vi "Detect Barcode.vi"() -> ()   [LabVIEW 2020]
doc: "Demonstrate the Barcode Detector"
uses:
  feature_detection/Barcode Detector/Detection.ctl
  feature_detection/Barcode Detector/Detection Region.ctl
  common/Image Point (Integer).ctl
  feature_detection/Barcode Detector/Barcode Detector.lvclass/Barcode Detector.ctl
  image/ARGB Colour.ctl
  image/Text Drawing Settings.ctl
  image/Font Face.ctl
  image/New Image (ARGB Preallocated).vi
  image/Copy Pixmap to Image (ARGB Flatten Mask).vi
  feature_detection/Barcode Detector/Detect Barcodes (ARGB).vi
  image/Draw Poly Lines (ARGB).vi
  image/Draw Text (ARGB).vi
  image/Draw Image to Picture (ARGB).vi
  image/New Image (ARGB Preallocated).vi/3321fa97-f432-4e1e-8db9-a0df79aed21b.vi
  image/ARGB Colour to U32 Pixel Value.vi
  image/Copy Pixmap to Image (ARGB Flatten Mask).vi/7d03ccf7-b889-4e8d-9f2a-57831e73dbde.vi
  feature_detection/Barcode Detector/Detect Barcodes (ARGB).vi/5cbfdd98-1063-43fc-ab47-121d1b6d8619.vi
  image/Draw Poly Lines (ARGB).vi/f4fe866f-059f-471d-887d-2797bd4b3b13.vi
  image/Draw Text (ARGB).vi/0015c4fc-6a12-4f82-815b-6c2f827f408b.vi
  image/Draw Image to Picture (ARGB).vi/8cd07b1b-062e-4fe4-9e87-2eb3dc89fe0e.vi
  image/FixPixmap.vi
  image/Default8bitColourMap.vi
  <vilib>/Utility/error.llb/Error Cluster From Error Code.vi
  image/image.lvlib
  feature_detection/Barcode Detector/Barcode Detector.lvclass
  common/common.lvlib
panel:
  out "Detections":T1[](array[typedef])
  out "Picture":picture
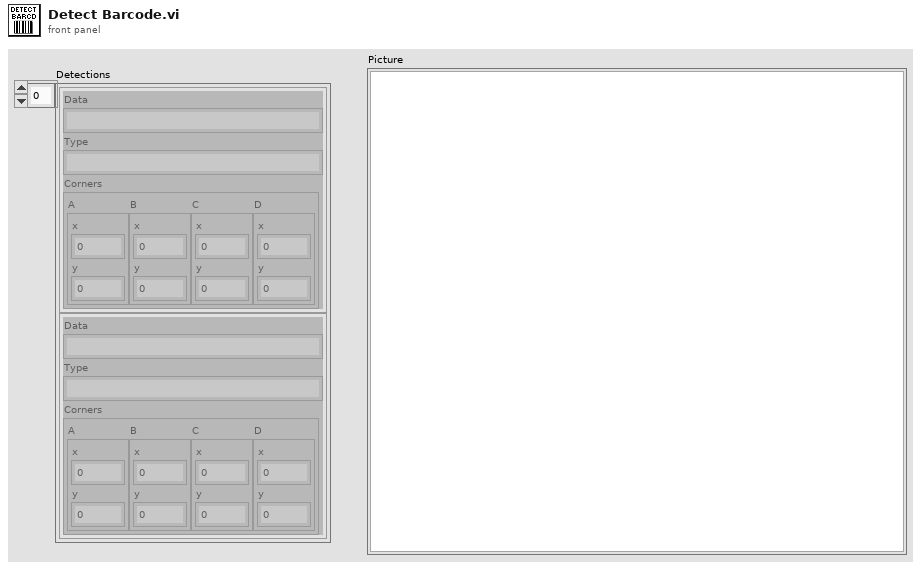
[diagram p1: front panel]
types:
  T1 = typedef "feature_detection.lvlib/Barcode Detector.lvclass/Detection.ctl" = cluster{"Data":string, "Type":string, "Corners":T2}
  T2 = typedef "feature_detection.lvlib/Barcode Detector.lvclass/Detection Region.ctl" = cluster{"A":T3, "B":T3, "C":T3, "D":T3}
  T3 = typedef "common.lvlib/Image Point (Integer).ctl" = cluster{"x":i32, "y":i32}
  T4 = typedef "image.lvlib/ARGB Image.ctl" = refnum<data-value>
  T5 = typedef "imagedata.ctl" = cluster{"image type":i32, "image depth":i32, "image":u8[], "mask":u8[], "colors":u32[], "Rectangle":cluster{"left":i16, "top":i16, "right":i16, "bottom":i16}}
  T6 = typedef "image.lvlib/Text Drawing Settings.ctl" = cluster{"OpenCV Font Face":T7, "Font Scale":dbl}
  T7 = typedef "image.lvlib/Font Face.ctl" = enum8{"FONT_HERSHEY_SIMPLEX", "FONT_HERSHEY_PLAIN", "FONT_HERSHEY_DUPLEX", "FONT_HERSHEY_COMPLEX", "FONT_HERSHEY_TRIPLEX", "FONT_HERSHEY_COMPLEX_SMALL", "FONT_HERSHEY_SCRIPT_SIMPLEX", "FONT_HERSHEY_SCRIPT_COMPLEX", "FONT_ITALIC"}
  T8 = typedef "image.lvlib/ARGB Colour.ctl" = cluster{"Alpha":u8, "RGB":u32}
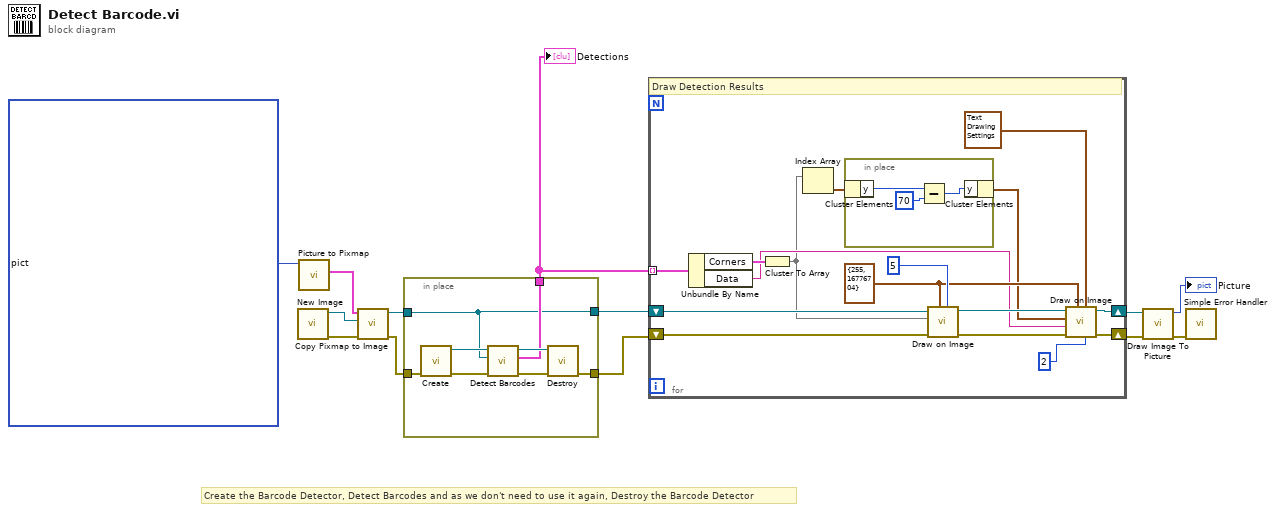
[diagram p0: block diagram]
diagram:
  # "Create the Barcode Detector, Detect Barcodes and as we don't need to use it again, Destroy the Barcode Detector"
  n1 = call-poly "New Image.vi"() -> ("error out"=w12:errorcluster, "ARGB Image"=w13:T4)  [unwired: 10 in]
  n2 = call <vilib>:"Picture to Pixmap.vi"("picture"=picture bytes[297327] ("new picture")) -> ("image data"=w4:T5)  [unwired: 9 in, 1 out]
  n3 = call-poly "Copy Pixmap to Image.vi"("error in (no error)"=w12, "ARGB Image Destination in"=w13, "Pixmap Image Data"=w4) -> ("error out"=w2:errorcluster, "ARGB Image Destination"=w5:T4)  [unwired: 7 in]
  n4 = in-place {
    in-place-border: [w19] -> w11
    in-place-border: [w18] -> w10
    in-place-border: w5 -> [w14]
    in-place-border: w2 -> [w16]
    in-place-border: [w14] -> w1
    n5 = call "Create.vi"("error in (no error)"=w16) -> ("error out"=w15:errorcluster, "Barcode Detector"=w17:refnum<class "Barcode Detector.lvclass">)  [unwired: 9 in]
    n6 = call-poly "Detect Barcodes.vi"("error in (no error)"=w15, "ARGB Image in"=w14, "Barcode Detector in"=w17) -> ("error out"=w20:errorcluster, "Detections"=w19:T1[], "Barcode Detector"=w21:refnum<class "Barcode Detector.lvclass">)  [unwired: 6 in]
    n7 = call "Destroy.vi"("error in (no error)"=w20, "Barcode Detector in"=w21) -> ("error out"=w18:errorcluster)  [unwired: 9 in]
  }
  "Detections" <- w11
  n8 = for {
    shift-right: [w29] -> w8
    shift-left: w1 -> [w37]
    tunnel: w11 -> [w36] mode=indexing
    shift-right: [w31] -> w9
    shift-left: w10 -> [w34]
    w28 = T8 {"Alpha"=255, "RGB"=16776704} ("ARGB Colour")
    # "Draw Detection Results"
    n9 = Unbundle By Name(w36) -> ("Corners"=w35:T2, "Data"=w27:string)
    n10 = Cluster To Array(cluster=w35) -> (array=w26:T3[])
    n11 = Index Array(array=w26) -> (element=w24:T3)  [unwired: 1 in]
    n12 = in-place {
      n13 = in-place-cluster #1(w24) -> ("y"=w40:i32)
      n14 = Subtract(x=w40, y=70 ("x")) -> (x-y=w39:i32)
      n15 = in-place-cluster #1("y"=w39) -> (w23:T3)
    }
    n16 = call-poly "Draw on Image.vi"("Thickness (Default: 1)"=5, "ARGB Colour"=w28, "error in (no error)"=w34, "Points"=w26, "ARGB Image in"=w37) -> ("error out"=w33:errorcluster, "ARGB Image"=w30:T4)  [unwired: 5 in]
    n17 = call-poly "Draw on Image.vi"("Thickness (Default: 1)"=2, "Text Drawing Settings (Default: Simplex)"=T6 {"OpenCV Font Face"=enum."FONT_HERSHEY_SIMPLEX", "Font Scale"=0.6}, "ARGB Colour"=w28, "error in (no error)"=w33, "Text"=w27, "Origin"=w23, "ARGB Image in"=w30) -> ("error out"=w31:errorcluster, "ARGB Image"=w29:T4)  [unwired: 3 in]
  }
  n18 = call-poly "Draw Image To Picture.vi"("error in (no error)"=w9, "ARGB Image Source in"=w8) -> ("error out"=w7:errorcluster, "Picture"=→"Picture":picture)  [unwired: 8 in]
  n19 = call <vilib>:"Simple Error Handler.vi"("error in (no error)"=w7) -> ()  [unwired: 4 in, 5 out]
